vi "FTW-HTTP-ParseResponseHeaders.vi"(5 "Response Headers":string, 11 "error in":errorcluster) -> (4 "HTTP Response Status Code":T1=100 items=["100 Continue"=100, "101 Switching Protocols"=101, "200 OK"=200, "201 Created"=201, "202 Accepted"=202, "203 Non-Authoritative Information"=203, "204 No Content"=204, "205 Reset Content"=205, "206 Partial Content"=206, "300 Multiple Choices"=300, "301 Moved Permanently"=301, "302 Found"=302, "303 See Other"=303, "304 Not Modified"=304, "305 Use Proxy"=305, "306 (Unused)"=306, "307 Temporary Redirect"=307, "400 Bad Request"=400, "401 Unauthorized"=401, "402 Payment Required"=402, "403 Forbidden"=403, "404 Not Found"=404, "405 Method Not Allowed"=405, "406 Not Acceptable"=406, "407 Proxy Authentication Required"=407, "408 Request Timeout"=408, "409 Conflict"=409, "410 Gone"=410, "411 Length Required"=411, "412 Precondition Failed"=412, "413 Request Entity Too Large"=413, "414 Request-URI Too Long"=414, "415 Unsupported Media Type"=415, "416 Requested Range Not Satisfiable"=416, "417 Expectation Failed"=417, "500 Internal Server Error"=500, "501 Not Implemented"=501, "502 Bad Gateway"=502, "503 Service Unavailable"=503, "504 Gateway Timeout"=504, "505 HTTP Version Not Supported"=505], 6 "HTTP Response Reason Phrase":string, 8 "Protocol":string, 10 "Headers":string, 15 "error out":errorcluster)   [LabVIEW 2013]
uses:
  FTW-HTTP-ResponseCode.ctl
panel:
  # "Inputs"
  # "Outputs"
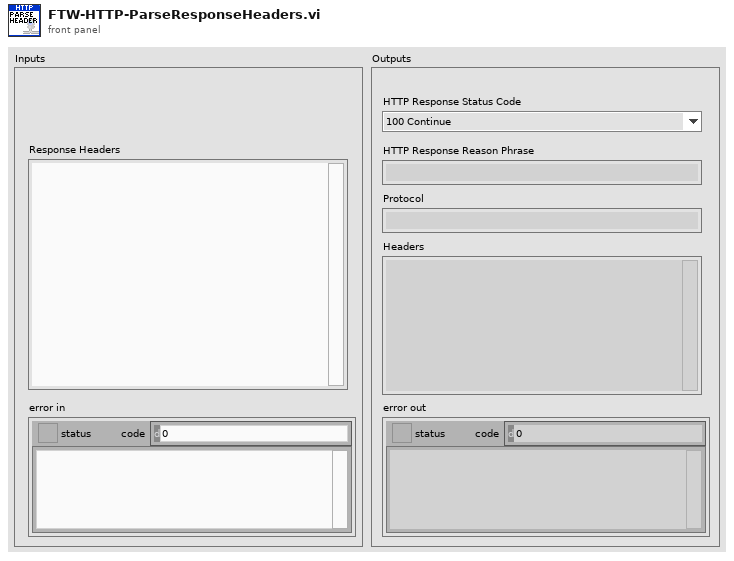
[diagram p1: front panel]
types:
  T1 = typedef "FTW-HTTP-ResponseCode.ctl" = i32
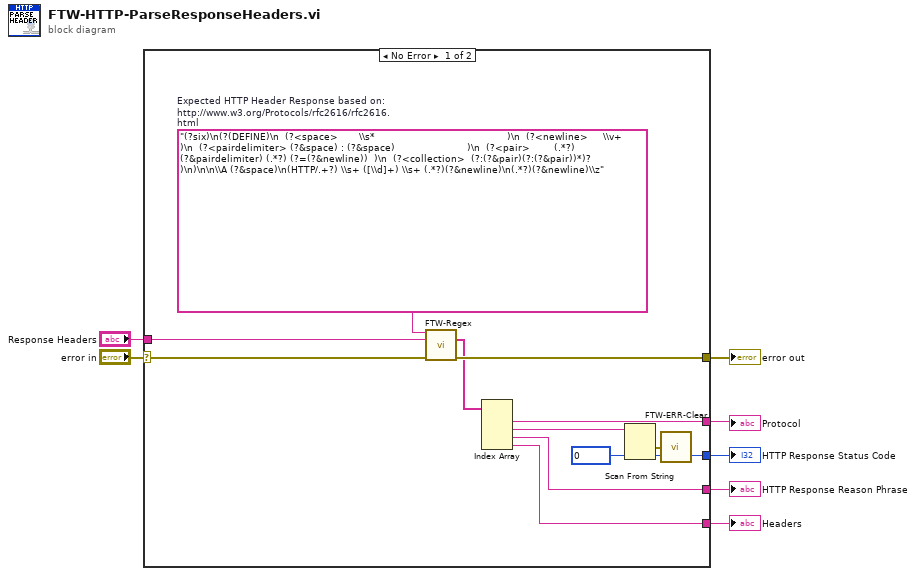
[diagram p0: block diagram]
diagram:
  n1 = case shown="No Error" "error in" {
    selector: "error in" -> [w18 w20]
    tunnel: [w17 w20] -> w7
    tunnel: "Response Headers" -> [w16 _]
    tunnel: [w14 _] -> w4
    tunnel: [w12 _] -> w3
    tunnel: [w11 _] -> w2
    tunnel: [w10 _] -> w1
    frame No Error {
      w9 = T1 0 items=["100 Continue"=100, "101 Switching Protocols"=101, "200 OK"=200, "201 Created"=201, "202 Accepted"=202, "203 Non-Authoritative Information"=203, "204 No Content"=204, "205 Reset Content"=205, "206 Partial Content"=206, "300 Multiple Choices"=300, "301 Moved Permanently"=301, "302 Found"=302, "303 See Other"=303, "304 Not Modified"=304, "305 Use Proxy"=305, "306 (Unused)"=306, "307 Temporary Redirect"=307, "400 Bad Request"=400, "401 Unauthorized"=401, "402 Payment Required"=402, "403 Forbidden"=403, "404 Not Found"=404, "405 Method Not Allowed"=405, "406 Not Acceptable"=406, "407 Proxy Authentication Required"=407, "408 Request Timeout"=408, "409 Conflict"=409, "410 Gone"=410, "411 Length Required"=411, "412 Precondition Failed"=412, "413 Request Entity Too Large"=413, "414 Request-URI Too Long"=414, "415 Unsupported Media Type"=415, "416 Requested Range Not Satisfiable"=416, "417 Expectation Failed"=417, "500 Internal Server Error"=500, "501 Not Implemented"=501, "502 Bad Gateway"=502, "503 Service Unavailable"=503, "504 Gateway Timeout"=504, "505 HTTP Version Not Supported"=505] ("HTTP Response Status Code")
      w19 = "(?six)\n(?(DEFINE)\n  (?<space>       \\s*                                            )\n  (?<newline>     \\v+                                            )\n  (?<pairdelimiter> (?&space) : (?&space)                        )\n  (?<pair>        (.*?) (?&pairdelimiter) (.*?) (?=(?&newline))  )\n  (?<collection>  (?:(?&pair)(?:(?&pair))*)?                     )\n)\n\n\\A (?&space)\n(HTTP/.+?) \\s+ ([\\d]+) \\s+ (.*?)(?&newline)\n(.*?)(?&newline)\\z"  # Expected HTTP Header Response based on: http://www.w3.org/Protocols/rfc2616/rfc2616.html
      n2 = call "FTW-Regex.vi"("Regular Expression"=w19, "Input String"=w16, "error in"=w18) -> ("Submatches"=w15:string[], "error out"=w17:errorcluster)  [unwired: 8 in, 3 out]
      n3 = Index Array(array=w15) -> (element #1=w14:string, element #2=w13:string, element #3=w10:string, element #4=w11:string)  [unwired: 4 in]
      n4 = Scan From String(input string=w13, default 1=w9) -> (error out=w8:errorcluster, output 1=w12:T1)  [unwired: 3 in, 2 out]
      n5 = call "FTW-ERR-Clear.vi"("error to snuff"=w8) -> ()  [unwired: 1 out]
    }
    frame Error {
    }
  }
  "error out" <- w7
  "Protocol" <- w4
  "Headers" <- w2
  "HTTP Response Status Code" <- w3
  "HTTP Response Reason Phrase" <- w1
